vi "Close.vi"(8 "error in (no error)":errorcluster, 11 "instrument handle":refnum<k15>) -> ()   [LabVIEW 2018]
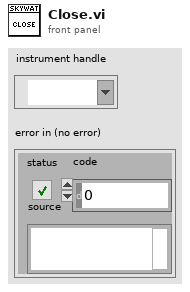
[diagram p1: front panel]
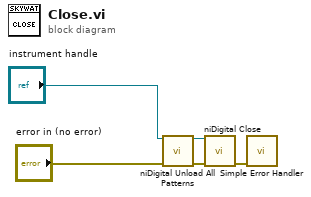
[diagram p0: block diagram]
diagram:
  n1 = call <instrlib>:"niDigital Unload All Patterns.vi"("instrument handle"="instrument handle", "error in"="error in (no error)") -> ("instrument handle out"=w2:refnum<k15>, "error out"=w3:errorcluster)  [unwired: 12 in]
  n2 = call <instrlib>:"niDigital Close.vi"("instrument handle"=w2, "error in"=w3) -> ("error out"=w1:errorcluster)  [unwired: 13 in]
  n3 = call <vilib>:"Simple Error Handler.vi"("error in (no error)"=w1) -> ()  [unwired: 4 in, 5 out]
